vi "move to target point_MFP3D.vi"(2 "PIS Close":bool, 8 "precision of nodes":i32=6, 9 "Litho Speed":dbl=5e-07 format="%#_6pm/s", 10 "Z SetPoint":dbl format="%#_6p", 11 "Target Point\n(  x      ,       y   )":dbl[](array[numeric])=[-5e-06, -5e-06] min=-4.5e-05 max=4.5e-05 step=1e-09 format="%#_6pm") -> ()   [LabVIEW 2019]
uses:
  Cypher XY LVDT Parameters_MFP3D.vi
panel:
  in  "?":bool
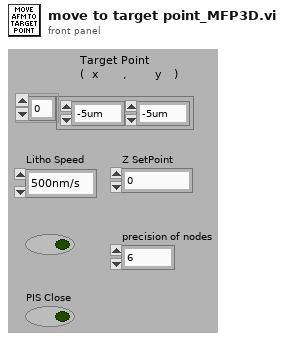
[diagram p1: front panel]
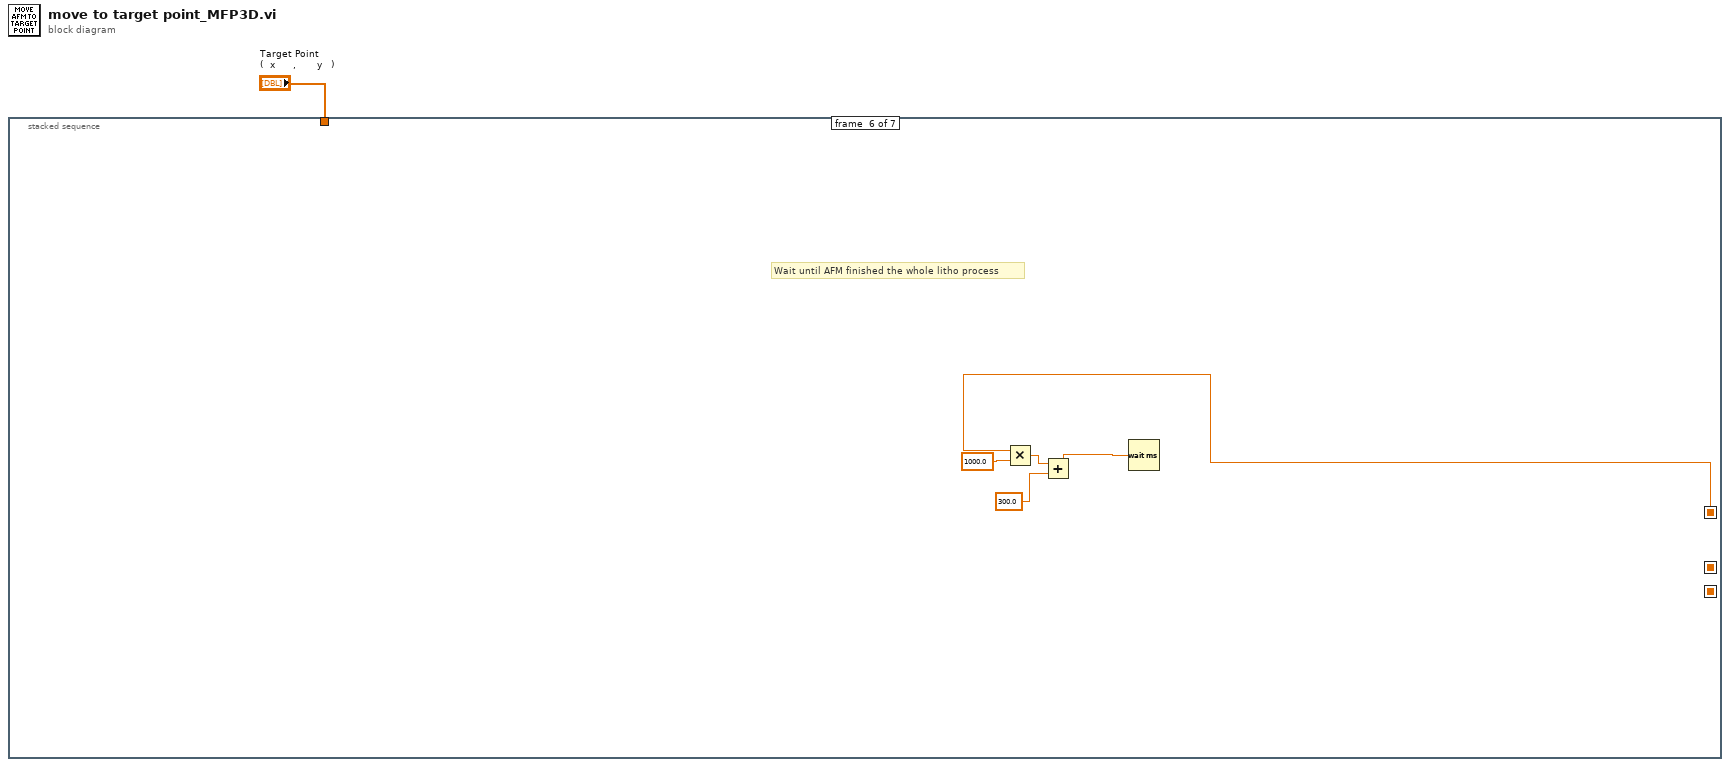
[diagram p0: block diagram]
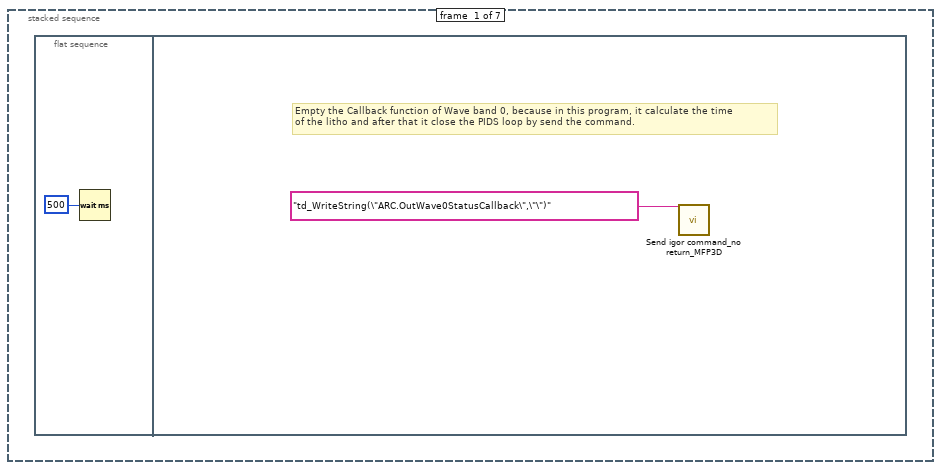
[diagram p2: hidden frame]
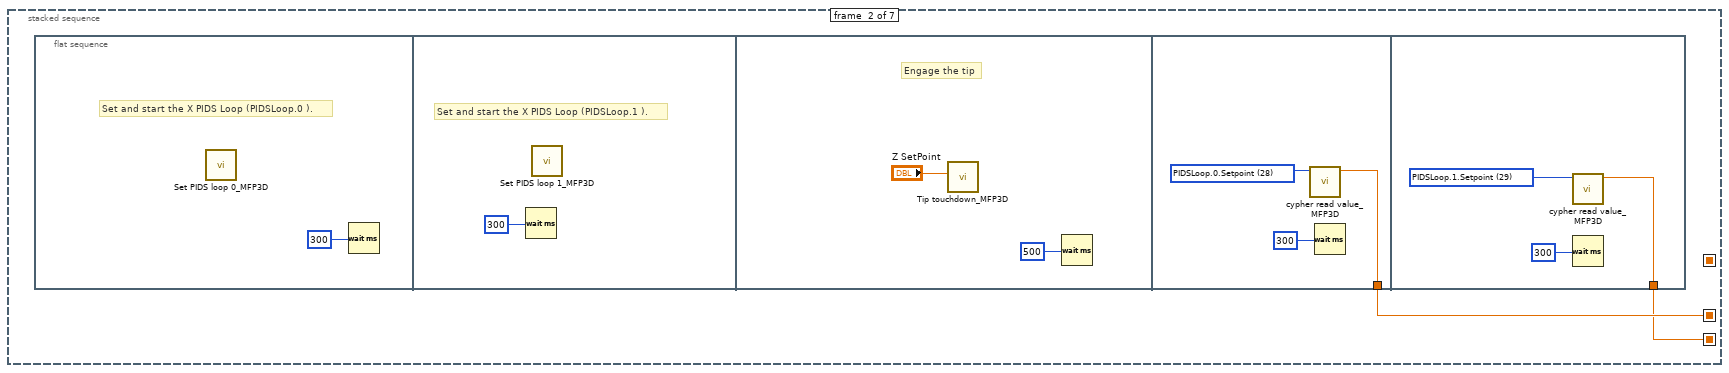
[diagram p3: hidden frame]
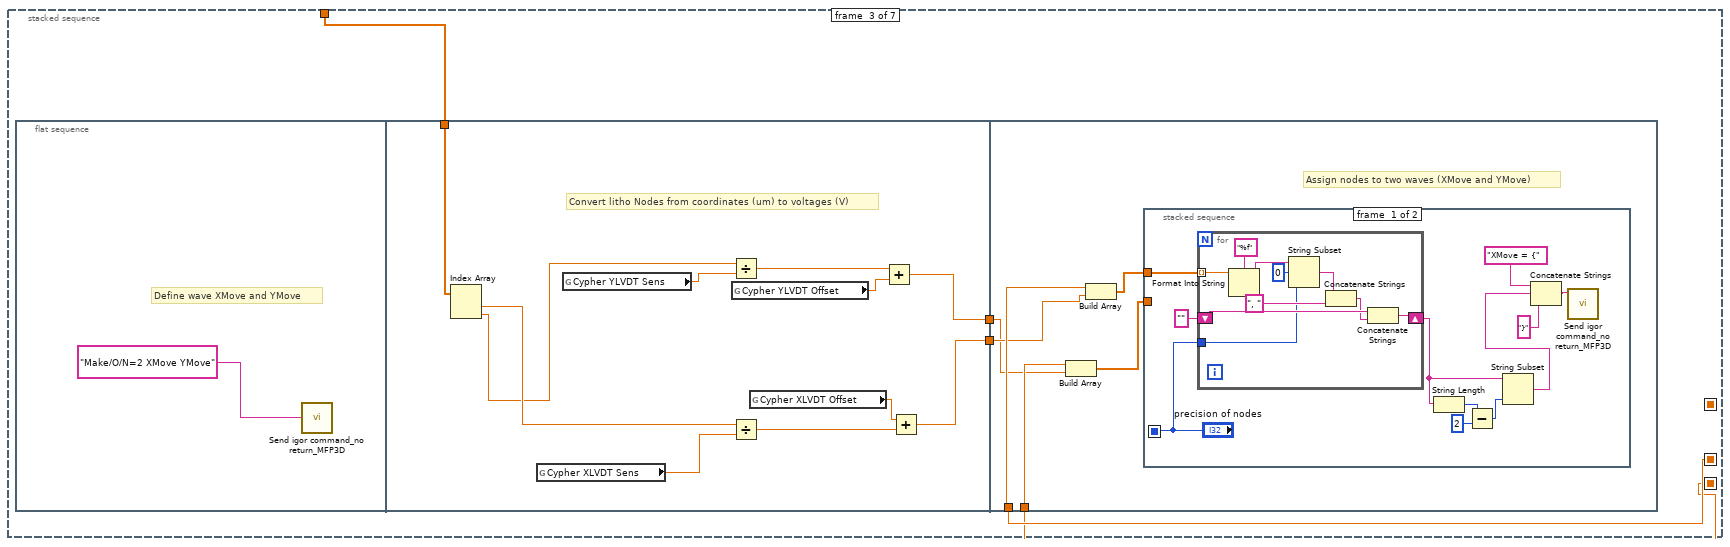
[diagram p4: hidden frame]
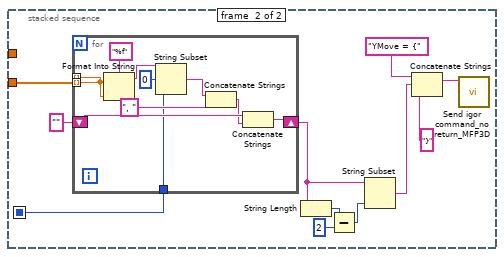
[diagram p5: hidden frame]
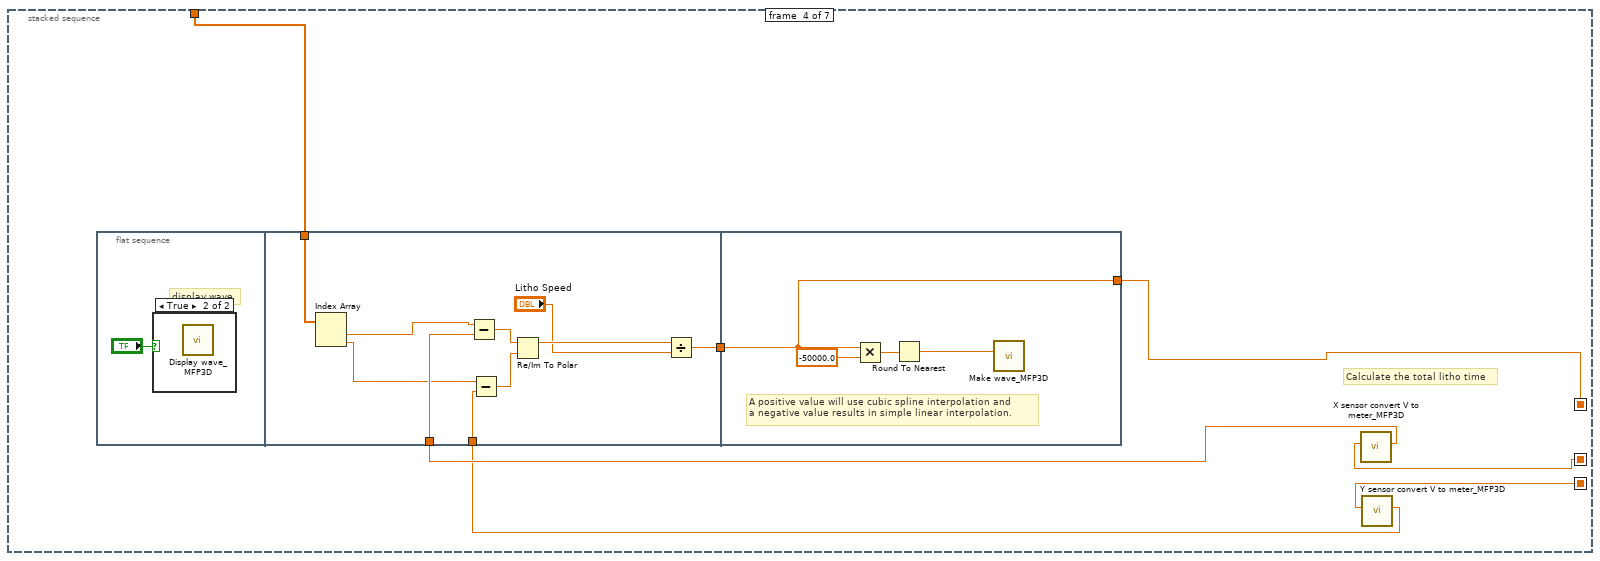
[diagram p6: hidden frame]
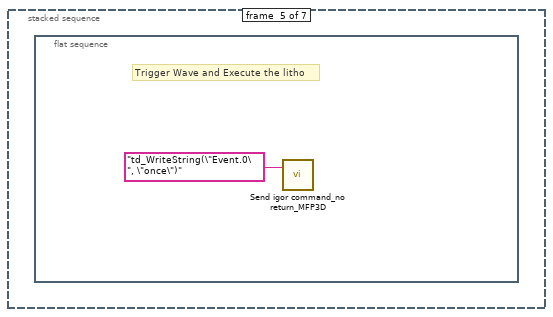
[diagram p8: hidden frame]
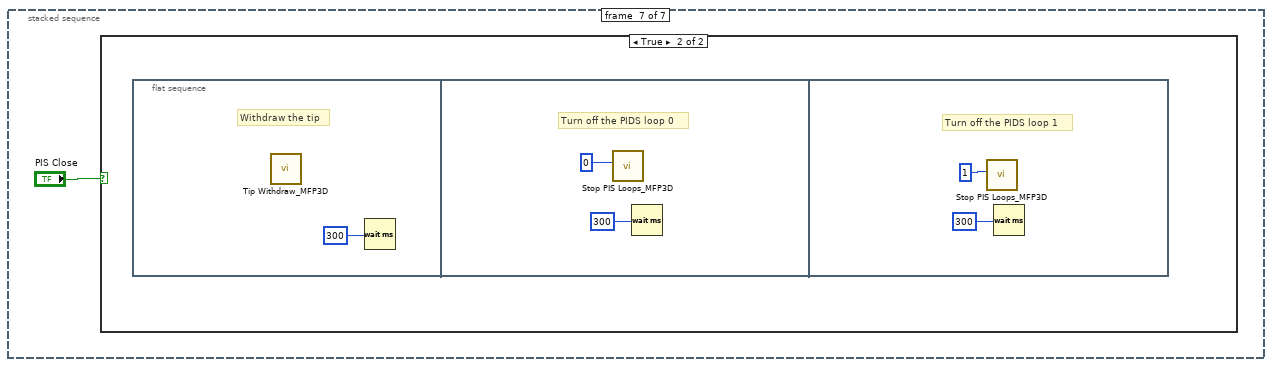
[diagram p9: hidden frame]
diagram:
  n1 = stacked-sequence {
    seq-local: [_ _ _ w86 _ _ _] -> [_ _ _ _ _ w107 _]
    seq-local: [_ w5 _ _ _ _ _] -> [_ _ w17 w85 _ _ _]
    seq-local: [_ w4 _ _ _ _ _] -> [_ _ w16 w84 _ _ _]
    tunnel: "Target Point\n(  x      ,       y   )" -> [_ _ w18 w83 _ _ _]
    frame #0 {
      n2 = flat-sequence {
        frame #0 {
          n3 = Wait (ms)(milliseconds to wait=u32 500) -> ()  [unwired: 1 out]
        }
        frame #1 {
          # "Empty the Callback function of Wave band 0, because in this program, it calculate the time \nof the litho and after that it close the PIDS loop by send the command."
          n4 = call "Send igor command_no return_MFP3D.vi"("Command"="td_WriteString(\"ARC.OutWave0StatusCallback\",\"\")") -> ()  [unwired: 11 out]
        }
      }
    }
    frame #1 {
      n5 = flat-sequence {
        tunnel: [w11] -> w5
        tunnel: [w14] -> w4
        frame #0 {
          # "Set and start the X PIDS Loop (PIDSLoop.0 )."
          n6 = call "Set PIDS loop 0_MFP3D.vi"() -> ()  [unwired: 12 in]
          n7 = Wait (ms)(milliseconds to wait=u32 300) -> ()  [unwired: 1 out]
        }
        frame #1 {
          # "Set and start the X PIDS Loop (PIDSLoop.1 )."
          n8 = Wait (ms)(milliseconds to wait=u32 300) -> ()  [unwired: 1 out]
          n9 = call "Set PIDS loop 1_MFP3D.vi"() -> ()  [unwired: 12 in]
        }
        frame #2 {
          # "Engage the tip"
          n10 = call "Tip touchdown_MFP3D.vi"("Z SetPoint"="Z SetPoint") -> ()  [unwired: 11 out]
          n11 = Wait (ms)(milliseconds to wait=u32 500) -> ()  [unwired: 1 out]
        }
        frame #3 {
          w12 = u16 28 items=["XSensor", "YSensor", "ZSensor", "InA", "InB", "InFast", "In_Amplitude1", "In_Amplitude2", "In_Phase1", "In_Phase2", "PiezoX", "PiezoY", "PiezoZ", "OutA", "OutB", "OutC", "DDS_Frequency1", "DDS_Frequency2", "DDS_Amplitude1", "DDS_Amplitude2", "DDS_DCOffset", "Laser_Sum", "Laser_Difference", "Laser_Lateral", "XLVDT Sensitivity", "YLVDT Sensitivity", "XLVDT Offset", "YLVDT Offset", "PIDSLoop.0.Setpoint", "PIDSLoop.1.Setpoint"] ("Input")
          n12 = call "cypher read value_MFP3D.vi"("Input"=w12) -> ("Result"=w11:dbl)  [unwired: 10 in]
          n13 = Wait (ms)(milliseconds to wait=u32 300) -> ()  [unwired: 1 out]
        }
        frame #4 {
          w15 = u16 29 items=["XSensor", "YSensor", "ZSensor", "InA", "InB", "InFast", "In_Amplitude1", "In_Amplitude2", "In_Phase1", "In_Phase2", "PiezoX", "PiezoY", "PiezoZ", "OutA", "OutB", "OutC", "DDS_Frequency1", "DDS_Frequency2", "DDS_Amplitude1", "DDS_Amplitude2", "DDS_DCOffset", "Laser_Sum", "Laser_Difference", "Laser_Lateral", "XLVDT Sensitivity", "YLVDT Sensitivity", "XLVDT Offset", "YLVDT Offset", "PIDSLoop.0.Setpoint", "PIDSLoop.1.Setpoint"] ("Input")
          n14 = call "cypher read value_MFP3D.vi"("Input"=w15) -> ("Result"=w14:dbl)  [unwired: 10 in]
          n15 = Wait (ms)(milliseconds to wait=u32 300) -> ()  [unwired: 1 out]
        }
      }
    }
    frame #2 {
      n16 = flat-sequence {
        tunnel: [w30] -> w20
        tunnel: [w29] -> w19
        tunnel: w18 -> [w28]
        tunnel: w20 -> [w34]
        tunnel: w19 -> [w36]
        tunnel: w17 -> [w38]
        tunnel: w16 -> [w37]
        frame #0 {
          # "Define wave XMove and YMove"
          n17 = call "Send igor command_no return_MFP3D.vi"("Command"="Make/O/N=2 XMove YMove") -> ()  [unwired: 11 out]
        }
        frame #1 {
          # "Convert litho Nodes from coordinates (um) to voltages (V)"
          n18 = Index Array(array=w28) -> (element #1=w27:dbl, element #2=w26:dbl)  [unwired: 2 in]
          n19 = global read "Cypher XY LVDT Parameters_MFP3D.vi" "Cypher XLVDT Sens"() -> (w22:dbl)
          n20 = global read "Cypher XY LVDT Parameters_MFP3D.vi" "Cypher YLVDT Sens"() -> (w25:dbl)
          n21 = Divide(x=w26, y=w25) -> (x/y=w31:dbl)
          n22 = Divide(x=w27, y=w22) -> (x/y=w32:dbl)
          n23 = global read "Cypher XY LVDT Parameters_MFP3D.vi" "Cypher YLVDT Offset"() -> (w24:dbl)
          n24 = global read "Cypher XY LVDT Parameters_MFP3D.vi" "Cypher XLVDT Offset"() -> (w23:dbl)
          n25 = Add(x=w31, y=w24) -> (x+y=w30:dbl)
          n26 = Add(x=w23, y=w32) -> (x+y=w29:dbl)
        }
        frame #2 {
          # "Assign nodes to two waves (XMove and YMove)"
          n27 = Build Array(w37, w34) -> (w33:dbl[])
          n28 = Build Array(w38, w36) -> (w35:dbl[])
          n29 = stacked-sequence {
            seq-local: ["precision of nodes" _] -> [_ w60]
            tunnel: w35 -> [w47 _]
            tunnel: w33 -> [_ w66]
            frame #0 {
              n30 = for {
                tunnel: w47 -> [w58] mode=indexing
                shift-right: [w56] -> w44
                shift-left: "" -> [w55]
                tunnel: "precision of nodes" -> [w50]
                n31 = Format Into String(format string="%f", w58) -> (resulting string=w52:string)  [unwired: 2 in, 1 out]
                n32 = String Subset(string=w52, offset (0)=0, length (rest)=w50) -> (substring=w51:string)
                n33 = Concatenate Strings(w51, ", " ("string")) -> (w54:string)
                n34 = Concatenate Strings(w55, w54) -> (w56:string)
              }
              n35 = String Length(string=w44) -> (length=w43:i32)
              n36 = Subtract(x=w43, y=2) -> (x-y=w41:i32)
              n37 = String Subset(string=w44, length (rest)=w41) -> (substring=w40:string)  [unwired: 1 in]
              n38 = Concatenate Strings("XMove = {" ("string"), w40, "}" ("string")) -> (w49:string)
              n39 = call "Send igor command_no return_MFP3D.vi"("Command"=w49) -> ()  [unwired: 11 out]
            }
            frame #1 {
              n40 = for {
                tunnel: [w75] -> _ mode=indexing
                shift-right: [w78] -> w61
                shift-left: "" -> [w77]
                tunnel: w66 -> [w75] mode=indexing
                tunnel: w60 -> [w71]
                n41 = Format Into String(format string="%f", w75) -> (resulting string=w74:string)  [unwired: 2 in, 1 out]
                n42 = String Subset(string=w74, offset (0)=0, length (rest)=w71) -> (substring=w72:string)
                n43 = Concatenate Strings(w72, ", " ("string")) -> (w76:string)
                n44 = Concatenate Strings(w77, w76) -> (w78:string)
              }
              n45 = String Length(string=w61) -> (length=w65:i32)
              n46 = Subtract(x=w65, y=2) -> (x-y=w63:i32)
              n47 = String Subset(string=w61, length (rest)=w63) -> (substring=w62:string)  [unwired: 1 in]
              n48 = Concatenate Strings("YMove = {" ("string"), w62, "}" ("string")) -> (w67:string)
              n49 = call "Send igor command_no return_MFP3D.vi"("Command"=w67) -> ()  [unwired: 11 out]
            }
          }
        }
      }
    }
    frame #3 {
      # "Calculate the total litho time"
      n50 = flat-sequence {
        tunnel: [w94] -> w87
        tunnel: w83 -> [w93]
        tunnel: w82 -> [w91]
        tunnel: w81 -> [w89]
        tunnel: w87 -> [w99]
        tunnel: [w99] -> w86
        frame #0 {
          # "display wave"
          n51 = case shown="True" "?" {
            frame False {
            }
            frame True {
              n52 = call "Display wave_MFP3D.vi"() -> ()  [unwired: 1 out]
            }
          }
        }
        frame #1 {
          n53 = Index Array(array=w93) -> (element #1=w92:dbl, element #2=w90:dbl)  [unwired: 2 in]
          n54 = Subtract(x=w92, y=w91) -> (x-y=w98:dbl)
          n55 = Subtract(x=w90, y=w89) -> (x-y=w97:dbl)
          n56 = Re/Im To Polar(2:w97, 3:w98) -> (1:w96:dbl)  [unwired: 1 out]
          n57 = Divide(x=w96, y="Litho Speed") -> (x/y=w94:dbl)
        }
        frame #2 {
          # "A positive value will use cubic spline interpolation and \na negative value results in simple linear interpolation."
          n58 = Multiply(x=w99, y=-50000.0) -> (x*y=w101:dbl)
          n59 = Round To Nearest(number=w101) -> (nearest integer value=w100:dbl)
          n60 = call "Make wave_MFP3D.vi"("Totalpoints"=w100) -> ()  [unwired: 11 out]
        }
      }
      n61 = call "X sensor convert V to meter_MFP3D.vi"("Sensor X Voltage"=w85) -> ("X coordinate"=w82:dbl)  [unwired: 10 in]
      n62 = call "Y sensor convert V to meter_MFP3D.vi"("Sensor Y Voltage"=w84) -> ("Y coordinate"=w81:dbl)  [unwired: 10 in]
    }
    frame #4 {
      n63 = flat-sequence {
        frame #0 {
          # "Trigger Wave and Execute the litho"
          n64 = call "Send igor command_no return_MFP3D.vi"("Command"="td_WriteString(\"Event.0\", \"once\")") -> ()  [unwired: 11 out]
        }
      }
    }
    frame #5 {
      # "Wait until AFM finished the whole litho process"
      n65 = Multiply(x=w107, y=1000.0) -> (x*y=w106:dbl)
      n66 = Add(x=w106, y=300.0) -> (x+y=w104:dbl)
      n67 = Wait (ms)(milliseconds to wait=w104) -> ()  [unwired: 1 out]
    }
    frame #6 {
      n68 = case shown="True" "PIS Close" {
        frame False {
        }
        frame True {
          n69 = flat-sequence {
            frame #0 {
              # "Withdraw the tip"
              n70 = call "Tip Withdraw_MFP3D.vi"() -> ()  [unwired: 1 in]
              n71 = Wait (ms)(milliseconds to wait=u32 300) -> ()  [unwired: 1 out]
            }
            frame #1 {
              # "Turn off the PIDS loop 0"
              n72 = call "Stop PIS Loops_MFP3D.vi"("PIS Loop Number (0-5)"=u32 0) -> ()  [unwired: 11 out]
              n73 = Wait (ms)(milliseconds to wait=u32 300) -> ()  [unwired: 1 out]
            }
            frame #2 {
              # "Turn off the PIDS loop 1"
              n74 = call "Stop PIS Loops_MFP3D.vi"("PIS Loop Number (0-5)"=u32 1) -> ()  [unwired: 11 out]
              n75 = Wait (ms)(milliseconds to wait=u32 300) -> ()  [unwired: 1 out]
            }
          }
        }
      }
    }
  }
